vi "HandleInput.vi"(8 "error in (no error)":errorcluster, 11 "TeleopInstruction":T1) -> (0 "error out":errorcluster, 2 "SkippedData?":bool, 3 "Time":u32)   [LabVIEW 2013]
uses:
  TeleopInstruction.ctl
  DriveData.ctl
  DoubleSolenoidAction.ctl
  CollectorWrapAction.ctl
  CollectorAction.ctl
  ShooterWrapperAction.ctl
  CatchAction.ctl
  QueueSubsystem.ctl
  QueueAction.ctl
  GetMainQueue.vi
  GetDriveQueue.vi
panel:
  in  "Deadzone":dbl=0.1
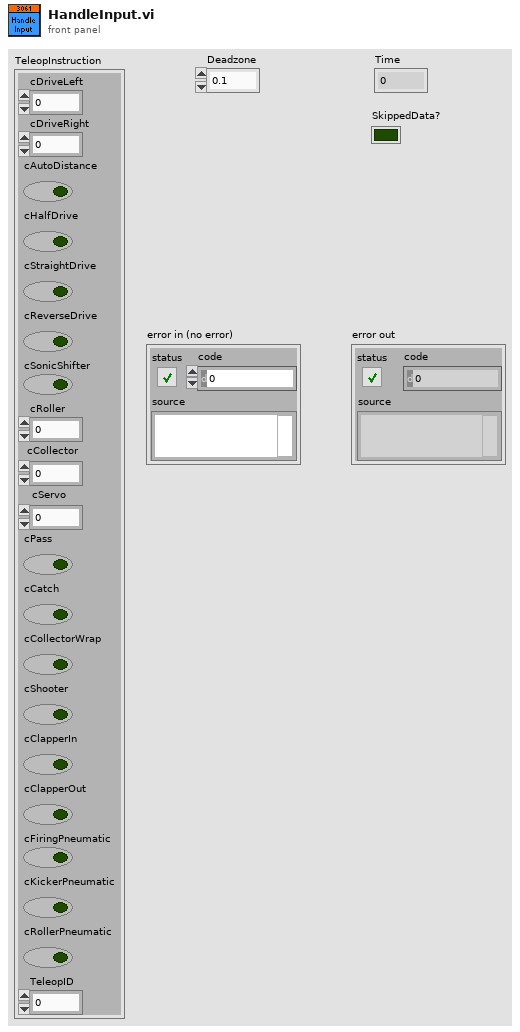
[diagram p1: front panel]
types:
  T1 = typedef "TeleopInstruction.ctl" = cluster{"cDriveLeft":dbl, "cDriveRight":dbl, "cAutoDistance":bool, "cHalfDrive":bool, "cStraightDrive":bool, "cReverseDrive":bool, "cSonicShifter":bool, "cRoller":dbl, "cCollector":dbl, "cServo":dbl, "cPass":bool, "cCatch":bool, "cCollectorWrap":bool, "cShooter":bool, "cClapperIn":bool, "cClapperOut":bool, "cFiringPneumatic":bool, "cKickerPneumatic":bool, "cRollerPneumatic":bool, "TeleopID":i32}
  T2 = typedef "CatchAction.ctl" = enum16{"PreCatch", "Catch", "Stop"}
  T3 = typedef "ShooterWrapperAction.ctl" = enum16{"Init", "CollectorDown", "CollectorUp"}
  T4 = typedef "CollectorAction.ctl" = enum16{"Init", "Raise", "Lower", "Stop", "GetStatus"}
  T5 = typedef "CollectorWrapAction.ctl" = enum16{"PreCollect", "Collect", "Stop"}
  T6 = typedef "DoubleSolenoidAction.ctl" = enum16{"Init", "Middle", "In", "Out"}
  T7 = typedef "DriveData.ctl" = cluster{"cDriveLeft":dbl, "cDriveRight":dbl, "cHalfDrive":bool, "cStraightDrive":bool, "cReverseDrive":bool}
  T8 = typedef "ServoAction.ctl" = enum16{"Init", "SetAngle", "GetAngle", "Lower", "Raise", "Disable"}
  T9 = typedef "RollerAction.ctl" = enum16{"Init", "Off", "Forward", "Reverse"}
  T10 = typedef "PassState.ctl" = enum16{"Pass", "Stop"}
  T11 = typedef "PassType.ctl" = enum16{"Ground", "Elevated"}
  T12 = typedef "QueueAction.ctl" = enum16{"Init", "SetValue", "Disable"}
  T13 = typedef "QueueSubsystem.ctl" = enum16{"Drive", "SonicShifter", "Kicker", "FiringPneumatic", "RollerPneumatic", "Clapper", "RollerMotor", "CollectorMotor", "Servo", "ShooterWrapper", "CollectorWrapper", "CatcherWrapper", "AutoDistance", "PassWrapper"}
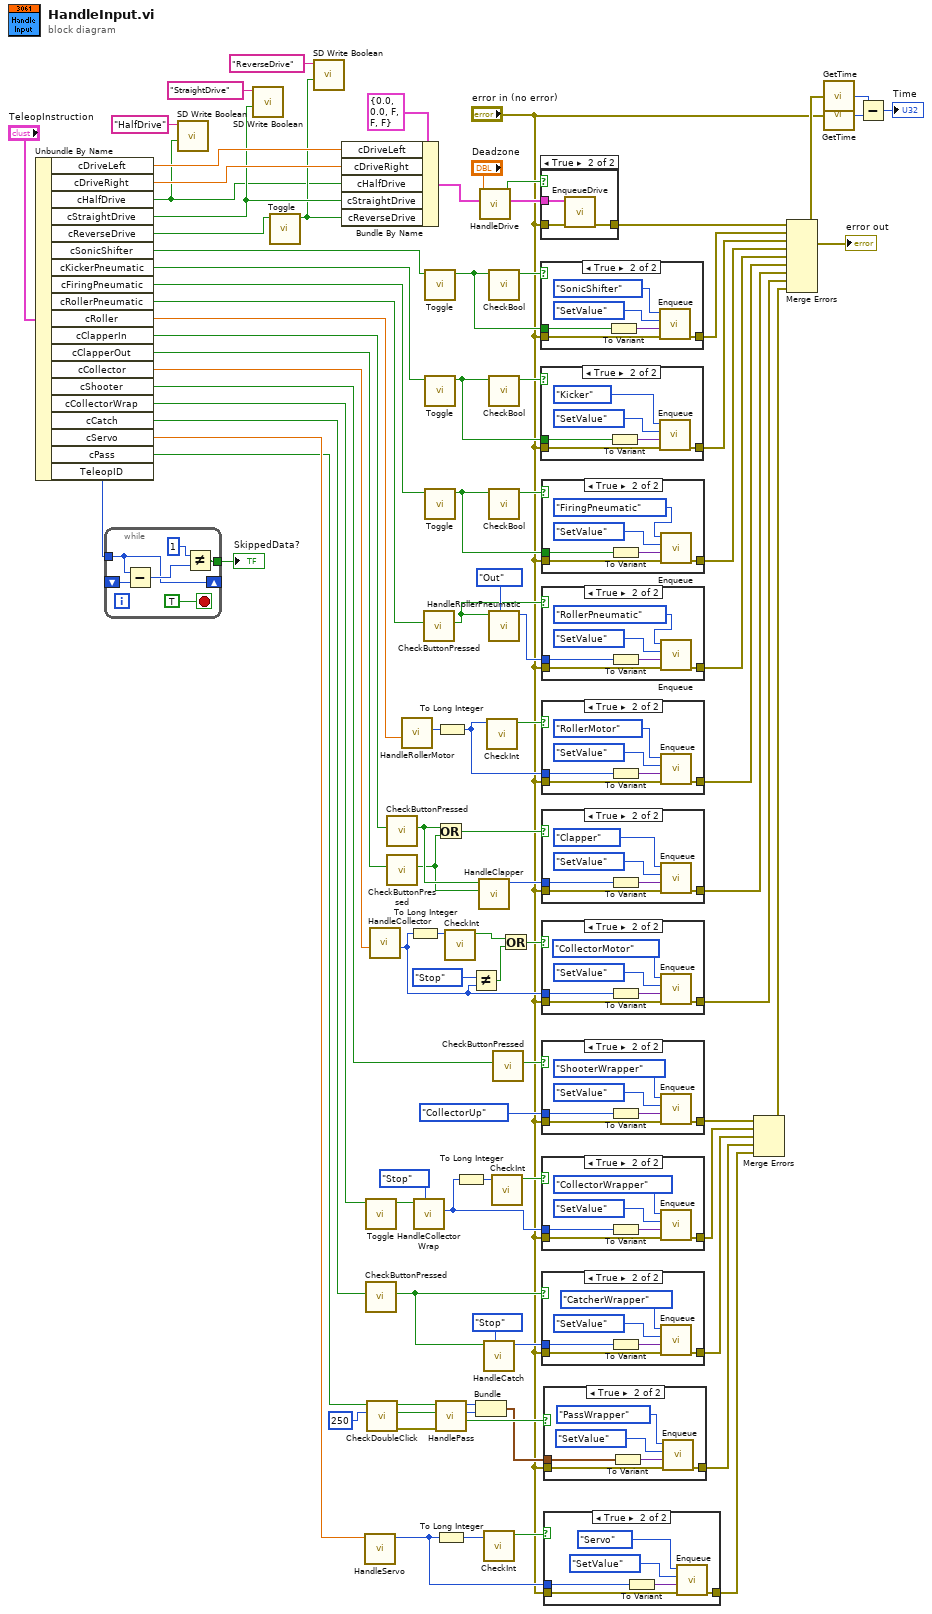
[diagram p0: block diagram]
diagram:
  n1 = Unbundle By Name("TeleopInstruction") -> ("cDriveLeft"=w85:dbl, "cDriveRight"=w84:dbl, "cHalfDrive"=w1:bool, "cStraightDrive"=w64:bool, "cReverseDrive"=w3:bool, "cSonicShifter"=w62:bool, "cKickerPneumatic"=w60:bool, "cFiringPneumatic"=w57:bool, "cRollerPneumatic"=w52:bool, "cRoller"=w43:dbl, "cClapperIn"=w48:bool, "cClapperOut"=w47:bool, "cCollector"=w35:dbl, "cShooter"=w28:bool, "cCollectorWrap"=w39:bool, "cCatch"=w24:bool, "cServo"=w19:dbl, "cPass"=w11:bool, "TeleopID"=w50:i32)
  n2 = while {
    tunnel: [w94] -> w68
    tunnel: w50 -> [w93]
    shift-right: [w93] -> _
    shift-left: _ -> [w97]
    stop <- TRUE stop-if-true
    n3 = Subtract(x=w93, y=w97) -> (x-y=w96:i32)
    n4 = Not Equal?(x=1, y=w96) -> (x != y?=w94:bool)
  }
  "SkippedData?" <- w68
  n5 = call <vilib>:"SD Write Boolean.vi"("Boolean"=w1, "Name"="HalfDrive") -> ()  [unwired: 8 in, 2 out]
  n6 = call <vilib>:"SD Write Boolean.vi"("Boolean"=w64, "Name"="StraightDrive") -> ()  [unwired: 8 in, 2 out]
  n7 = call "Toggle.vi"("Input"=w3) -> ("Output"=w2:bool)  [unwired: 10 in]
  n8 = call <vilib>:"SD Write Boolean.vi"("Boolean"=w2, "Name"="ReverseDrive") -> ()  [unwired: 8 in, 2 out]
  n9 = Bundle By Name(cluster=T7 {"cDriveLeft"=0.0, "cDriveRight"=0.0, "cHalfDrive"=FALSE, "cStraightDrive"=FALSE, "cReverseDrive"=FALSE} ("DriveInstruction"), "cDriveLeft"=w85, "cDriveRight"=w84, "cHalfDrive"=w1, "cStraightDrive"=w64, "cReverseDrive"=w2) -> (w82:T7)
  n10 = call "HandleServo.vi"("DPadValue"=w19) -> ("Action"=w16:T8)  [unwired: 10 in]
  n11 = call "Toggle.vi"("Input"=w39) -> ("Output"=w71:bool)  [unwired: 10 in]
  n12 = call "CheckButtonPressed.vi"("Button"=w24) -> ("Pressed?"=w21:bool)  [unwired: 9 in, 1 out]
  n13 = call "CheckDoubleClick.vi"("Timeout"=u32 250, "cPass"=w11) -> ("error out"=w13:errorcluster, "Perform?"=w14:bool, "Double Click?"=w15:bool)  [unwired: 7 in]
  n14 = call "HandleCollector.vi"("JoystickValue"=w35) -> ("CollectorEnum Input"=w34:T4)  [unwired: 9 in, 1 out]
  n15 = call "CheckButtonPressed.vi"("Button"=w48) -> ("Pressed?"=w45:bool)  [unwired: 9 in, 1 out]
  n16 = call "CheckButtonPressed.vi"("Button"=w47) -> ("Pressed?"=w44:bool)  [unwired: 9 in, 1 out]
  n17 = call "HandleRollerMotor.vi"("JoystickValue"=w43) -> ("StateOut"=w42:T9)  [unwired: 9 in, 1 out]
  n18 = To Long Integer(number=w34) -> (32bit integer=w36:i32)
  n19 = call "HandleCollectorWrap.vi"("InitState"=CollectorWrapAction."Stop" ("Action"), "Toggle?"=w71) -> ("State"=w69:T5)  [unwired: 8 in, 1 out]
  n20 = call "CheckButtonPressed.vi"("Button"=w52) -> ("Pressed?"=w51:bool)  [unwired: 9 in, 1 out]
  n21 = call "Toggle.vi"("Input"=w62) -> ("Output"=w61:bool)  [unwired: 10 in]
  n22 = call "Toggle.vi"("Input"=w60) -> ("Output"=w58:bool)  [unwired: 10 in]
  n23 = call "Toggle.vi"("Input"=w57) -> ("Output"=w55:bool)  [unwired: 10 in]
  n24 = Or(x=w45, y=w44) -> (x .or. y?=w46:bool)
  n25 = call "HandlePass.vi"("error in (no error)"=w13, "Perform?"=w14, "DoubleClick?"=w15) -> ("Call?"=w10:bool, "PassState"=w8:T10, "PassType"=w9:T11)  [unwired: 5 in, 1 out]
  n26 = To Long Integer(number=w16) -> (32bit integer=w18:i32)
  n27 = To Long Integer(number=w42) -> (32bit integer=w40:i32)
  n28 = call "CheckInt.vi"("Integer"=w36) -> ("Changed?"=w31:bool)  [unwired: 10 in]
  n29 = To Long Integer(number=w69) -> (32bit integer=w70:i32)
  n30 = Not Equal?(x=CollectorAction."Stop", y=w34) -> (x != y?=w30:bool)
  n31 = Bundle("PassType"=w9, "PassState"=w8) -> (w7:cluster{"PassType":T11, "PassState":T10})  [unwired: 1 in]
  n32 = call "HandleClapper.vi"("ClapperOut"=w44, "ClapperIn"=w45) -> ("State"=w49:T6)  [unwired: 8 in, 1 out]
  n33 = call "HandleDrive.vi"("DriveInstruction"=w82, "Deadzone"="Deadzone") -> ("DriveInstruction"=w83:T7, "Enqueue?"=w87:bool)  [unwired: 8 in]
  n34 = call "HandleCatch.vi"("InitState"=CatchAction."Stop", "Toggle?"=w21) -> ("State"=w23:T2)  [unwired: 8 in, 1 out]
  n35 = call "CheckInt.vi"("Integer"=w18) -> ("Changed?"=w17:bool)  [unwired: 10 in]
  n36 = call "CheckInt.vi"("Integer"=w40) -> ("Changed?"=w41:bool)  [unwired: 10 in]
  n37 = call "CheckBool.vi"("Input Boolean"=w61) -> ("Boolean Changed?"=w63:bool)  [unwired: 10 in]
  n38 = call "CheckBool.vi"("Input Boolean"=w58) -> ("Boolean Changed?"=w59:bool)  [unwired: 10 in]
  n39 = call "CheckBool.vi"("Input Boolean"=w55) -> ("Boolean Changed?"=w56:bool)  [unwired: 10 in]
  n40 = call "HandleRollerPneumatic.vi"("InitState"=DoubleSolenoidAction."Out", "Toggle?"=w51) -> ("State"=w54:T6)  [unwired: 8 in, 1 out]
  n41 = call "CheckInt.vi"("Integer"=w70) -> ("Changed?"=w72:bool)  [unwired: 10 in]
  n42 = call "CheckButtonPressed.vi"("Button"=w28) -> ("Pressed?"=w29:bool)  [unwired: 9 in, 1 out]
  n43 = Or(x=w31, y=w30) -> (x .or. y?=w32:bool)
  n44 = case shown="True" w87 {
    tunnel: [w99 w102] -> w81
    tunnel: "error in (no error)" -> [w99 w101]
    tunnel: w83 -> [_ w100]
    frame False {
    }
    frame True {
      n45 = call "EnqueueDrive.vi"("error in (no error)"=w101, "DriveInstruction"=w100) -> ("error out"=w102:errorcluster)  [unwired: 9 in]
    }
  }
  n46 = case shown="True" w63 {
    tunnel: "error in (no error)" -> [w103 w109]
    tunnel: [w103 w108] -> w80
    tunnel: w61 -> [_ w104]
    frame False {
    }
    frame True {
      n47 = To Variant(anything=w104) -> (Variant=w105:variant)
      n48 = call "Enqueue.vi"("error in (no error)"=w109, "Data"=w105, "Action"=QueueAction."SetValue", "Subsystem"=QueueSubsystem."SonicShifter") -> ("error out"=w108:errorcluster)  [unwired: 7 in]
    }
  }
  n49 = case shown="True" w59 {
    tunnel: w58 -> [_ w112]
    tunnel: "error in (no error)" -> [w110 w116]
    tunnel: [w110 w111] -> w78
    frame False {
    }
    frame True {
      n50 = To Variant(anything=w112) -> (Variant=w113:variant)
      n51 = call "Enqueue.vi"("error in (no error)"=w116, "Data"=w113, "Action"=QueueAction."SetValue", "Subsystem"=QueueSubsystem."Kicker") -> ("error out"=w111:errorcluster)  [unwired: 7 in]
    }
  }
  n52 = case shown="True" w56 {
    tunnel: w55 -> [_ w119]
    tunnel: "error in (no error)" -> [w117 w123]
    tunnel: [w117 w118] -> w77
    frame False {
    }
    frame True {
      n53 = To Variant(anything=w119) -> (Variant=w120:variant)
      n54 = call "Enqueue.vi"("error in (no error)"=w123, "Data"=w120, "Action"=QueueAction."SetValue", "Subsystem"=QueueSubsystem."FiringPneumatic") -> ("error out"=w118:errorcluster)  [unwired: 7 in]
    }
  }
  n55 = case shown="True" w51 {
    tunnel: w54 -> [_ w126]
    tunnel: "error in (no error)" -> [w124 w130]
    tunnel: [w124 w125] -> w76
    frame False {
    }
    frame True {
      n56 = To Variant(anything=w126) -> (Variant=w127:variant)
      n57 = call "Enqueue.vi"("error in (no error)"=w130, "Data"=w127, "Action"=QueueAction."SetValue", "Subsystem"=QueueSubsystem."RollerPneumatic") -> ("error out"=w125:errorcluster)  [unwired: 7 in]
    }
  }
  n58 = case shown="True" w41 {
    tunnel: "error in (no error)" -> [w131 w137]
    tunnel: [w131 w133] -> w75
    tunnel: w40 -> [_ w132]
    frame False {
    }
    frame True {
      n59 = To Variant(anything=w132) -> (Variant=w134:variant)
      n60 = call "Enqueue.vi"("error in (no error)"=w137, "Data"=w134, "Action"=QueueAction."SetValue", "Subsystem"=QueueSubsystem."RollerMotor") -> ("error out"=w133:errorcluster)  [unwired: 7 in]
    }
  }
  n61 = case shown="True" w46 {
    tunnel: "error in (no error)" -> [w138 w144]
    tunnel: [w138 w140] -> w74
    tunnel: w49 -> [_ w139]
    frame False {
    }
    frame True {
      n62 = To Variant(anything=w139) -> (Variant=w141:variant)
      n63 = call "Enqueue.vi"("error in (no error)"=w144, "Data"=w141, "Action"=QueueAction."SetValue", "Subsystem"=QueueSubsystem."Clapper") -> ("error out"=w140:errorcluster)  [unwired: 7 in]
    }
  }
  n64 = case shown="True" w32 {
    tunnel: "error in (no error)" -> [w145 w151]
    tunnel: [w145 w147] -> w37
    tunnel: w34 -> [_ w146]
    frame False {
    }
    frame True {
      n65 = To Variant(anything=w146) -> (Variant=w148:variant)
      n66 = call "Enqueue.vi"("error in (no error)"=w151, "Data"=w148, "Action"=QueueAction."SetValue", "Subsystem"=QueueSubsystem."CollectorMotor") -> ("error out"=w147:errorcluster)  [unwired: 7 in]
    }
  }
  n67 = case shown="True" w29 {
    tunnel: ShooterWrapperAction."CollectorUp" ("Operation") -> [_ w154]
    tunnel: "error in (no error)" -> [w152 w158]
    tunnel: [w152 w153] -> w26
    frame False {
    }
    frame True {
      n68 = To Variant(anything=w154) -> (Variant=w155:variant)
      n69 = call "Enqueue.vi"("error in (no error)"=w158, "Data"=w155, "Action"=QueueAction."SetValue", "Subsystem"=QueueSubsystem."ShooterWrapper") -> ("error out"=w153:errorcluster)  [unwired: 7 in]
    }
  }
  n70 = case shown="True" w72 {
    tunnel: w69 -> [_ w161]
    tunnel: "error in (no error)" -> [w159 w165]
    tunnel: [w159 w160] -> w38
    frame False {
    }
    frame True {
      n71 = To Variant(anything=w161) -> (Variant=w162:variant)
      n72 = call "Enqueue.vi"("error in (no error)"=w165, "Data"=w162, "Action"=QueueAction."SetValue", "Subsystem"=QueueSubsystem."CollectorWrapper") -> ("error out"=w160:errorcluster)  [unwired: 7 in]
    }
  }
  n73 = case shown="True" w21 {
    tunnel: w23 -> [_ w168]
    tunnel: "error in (no error)" -> [w166 w172]
    tunnel: [w166 w167] -> w20
    frame False {
    }
    frame True {
      n74 = To Variant(anything=w168) -> (Variant=w169:variant)
      n75 = call "Enqueue.vi"("error in (no error)"=w172, "Data"=w169, "Action"=QueueAction."SetValue", "Subsystem"=QueueSubsystem."CatcherWrapper") -> ("error out"=w167:errorcluster)  [unwired: 7 in]
    }
  }
  n76 = case shown="True" w10 {
    tunnel: w7 -> [_ w175]
    tunnel: "error in (no error)" -> [w173 w179]
    tunnel: [w173 w174] -> w4
    frame False {
    }
    frame True {
      n77 = To Variant(anything=w175) -> (Variant=w176:variant)
      n78 = call "Enqueue.vi"("error in (no error)"=w179, "Data"=w176, "Action"=QueueAction."SetValue", "Subsystem"=QueueSubsystem."PassWrapper") -> ("error out"=w174:errorcluster)  [unwired: 7 in]
    }
  }
  n79 = case shown="True" w17 {
    tunnel: w16 -> [_ w182]
    tunnel: "error in (no error)" -> [w180 w186]
    tunnel: [w180 w181] -> w5
    frame False {
    }
    frame True {
      n80 = To Variant(anything=w182) -> (Variant=w183:variant)
      n81 = call "Enqueue.vi"("error in (no error)"=w186, "Data"=w183, "Action"=QueueAction."SetValue", "Subsystem"=QueueSubsystem."Servo") -> ("error out"=w181:errorcluster)  [unwired: 7 in]
    }
  }
  n82 = Merge Errors(w26, w38, w20, w4, w5) -> (w25:errorcluster)
  n83 = Merge Errors(w81, w80, w78, w77, w76, w75, w74, w37, w25) -> (w79:errorcluster)
  "error out" <- w79
  n84 = call "GetTime.vi"("error in"=w79) -> ("Time"=w91:u32)
  n85 = call "GetTime.vi"("error in"="error in (no error)") -> ("Time"=w90:u32)
  n86 = Subtract(x=w91, y=w90) -> (x-y=→"Time":u32)
